vi "Read LLP Packet Word Cache.vi"(0 "state in":T1, 5 "bytes to read":fxp<+,4,4>) -> (4 "state out":T1, 6 "cached bytes":u8[](array[numeric]))   [LabVIEW 2020, in "GettingStarted_Common_148X_FPGA.lvlib"]
uses:
  <instrlib>/FlexRIO/CSI-2/v2/FPGA/Types/Deserialize LLP Packet State Data.ctl
  <instrlib>/FlexRIO/CSI-2/v2/FPGA/Types/FPGA LLP Packet Timestamp.ctl
  <instrlib>/FlexRIO/CSI-2/v2/FPGA/Types/Timestamp ID.ctl
  <instrlib>/FlexRIO/CSI-2/v2/FPGA/Types/Deserialize LLP Packet State.ctl
  GettingStarted_Common_148X_FPGA.lvlib
  <instrlib>/FlexRIO/CSI-2/v2/FPGA/NI CSI-2 API FPGA v2.lvlib
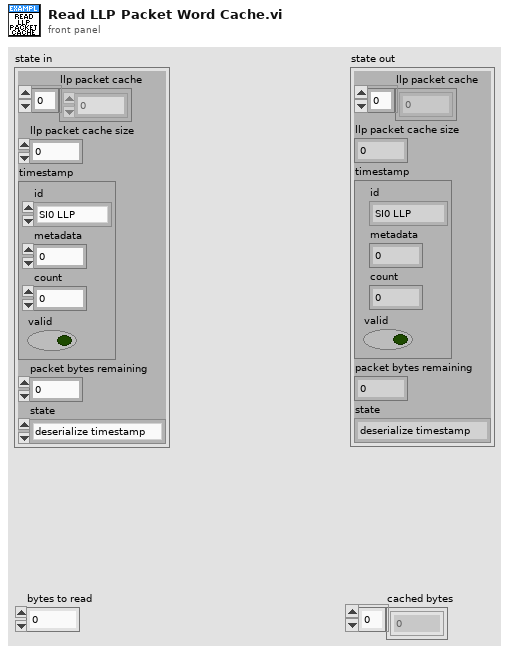
[diagram p1: front panel]
types:
  T1 = typedef "NI CSI-2 API FPGA v2.lvlib/Deserialize LLP Packet State Data.ctl" = cluster{"llp packet cache":u8[], "llp packet cache size":fxp<+,4,4>, "timestamp":T2, "packet bytes remaining":fxp<+,17,17>, "state":T4}
  T2 = typedef "NI CSI-2 API FPGA v2.lvlib/FPGA LLP Packet Timestamp.ctl" = cluster{"valid":bool, "count":fxp<+,50,50>, "id":T3, "metadata":u8}
  T3 = typedef "NI CSI-2 API FPGA v2.lvlib/Timestamp ID.ctl" = enum8{"SI0 LLP", "SI1 LLP", "SI2 LLP", "SI3 LLP", "SI4 LLP", "SI5 LLP", "SI6 LLP", "SI7 LLP", "SO0 LLP", "SO1 LLP", "SO2 LLP", "SO3 LLP", "SO4 LLP", "SO5 LLP", "SO6 LLP", "SO7 LLP", "Ser0 GPIO Bank", "Ser1 GPIO Bank", "Ser2 GPIO Bank", "Ser3 GPIO Bank", "Ser4 GPIO Bank", "Ser5 GPIO Bank", "Ser6 GPIO Bank", "Ser7 GPIO Bank", "Des0 GPIO Bank", "Des1 GPIO Bank", "Des2 GPIO Bank", "Des3 GPIO Bank", "Des4 GPIO Bank", "Des5 GPIO Bank", "Des6 GPIO Bank", "Des7 GPIO Bank", "User0", "User1", "User2", "User3", "User4", "User5", "User6", "User7", "User8", "User9", "User10", "User11", "User12", "User13", "User14", "User15", "User16", "User17", "User18", "User19", "User20", "User21", "User22", "User23", "User24", "User25", "User26", "User27", "User28", "User29", "User30", "User31"}
  T4 = typedef "NI CSI-2 API FPGA v2.lvlib/Deserialize LLP Packet State.ctl" = enum8{"deserialize timestamp", "deserialize size and header", "deserialize payload"}
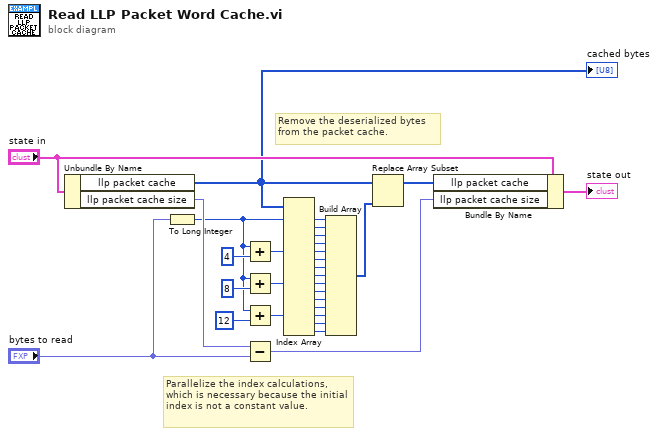
[diagram p0: block diagram]
diagram:
  # "Parallelize the index calculations, which is necessary because the initial index is not a constant value."
  # "Remove the deserialized bytes \nfrom the packet cache."
  n1 = Unbundle By Name("state in") -> ("llp packet cache"=w13:u8[], "llp packet cache size"=w25:fxp<+,4,4>)
  "cached bytes" <- w13
  n2 = To Long Integer(number="bytes to read") -> (32bit integer=w1:i32)
  n3 = Add(x=w1, y=4) -> (x+y=w12:i32)
  n4 = Add(x=w1, y=8) -> (x+y=w11:i32)
  n5 = Add(x=w1, y=12) -> (x+y=w2:i32)
  n6 = Subtract(x=w25, y="bytes to read") -> (x-y=w23:fxp<+,4,4>)
  n7 = Index Array(array=w13, index #1=w1, index #5=w12, index #9=w11, index #13=w2) -> (element #1=w20:u8, element #2=w19:u8, element #3=w18:u8, element #4=w17:u8, element #5=w16:u8, element #6=w15:u8, element #7=w14:u8, element #8=w29:u8, element #9=w28:u8, element #10=w27:u8, element #11=w26:u8, element #12=w7:u8, element #13=w6:u8, element #14=w5:u8, element #15=w4:u8)  [unwired: 11 in]
  n8 = Build Array(w20, w19, w18, w17, w16, w15, w14, w29, w28, w27, w26, w7, w6, w5, w4) -> (w21:u8[])
  n9 = Replace Array Subset(array=w13, new element=w21) -> (w22:u8[])  [unwired: 1 in]
  n10 = Bundle By Name(cluster="state in", "llp packet cache"=w22, "llp packet cache size"=w23) -> (→"state out":T1)
